vi "Module Loop.vi"(8 "error in (no error)":errorcluster, 11 "DAQmxAO in":refnum<class "DAQmxAO.lvclass">) -> (0 "error out":errorcluster, 3 "DAQmxAO out":refnum<class "DAQmxAO.lvclass">)   [LabVIEW 2023, in "VolatusDAQ.lvlib" / "DAQmxAO.lvclass"]
uses:
  DAQmxAO.lvclass
  DAQmxAO.lvclass/DAQmxAO.ctl
  Volatus/Module/Module.lvclass
  Volatus/MessageQ/MessageQ.lvclass/MessageQ.ctl
  messages/CmdAnalog/Class/Msg.lvclass/Msg.ctl
  Volatus/Module/Module.lvclass/Module.ctl
  messages/CmdAnalog/Data.ctl
  VolatusData/Scaling/Scaling.lvclass/Scaling.ctl
  messages/CmdAnalogMultiple/Class/Msg.lvclass
  messages/CmdAnalogMultiple/Class/Msg.lvclass/Msg.ctl
  <vilib>/DAQmx/write.llb/DAQmx Write (Analog 1D DBL NChan 1Samp).vi
  VolatusData/Send New Data (Array).vi
  Volatus/Module/Self Q.vi
  Volatus/MessageQ/Send.vi
  VolatusData/Scaling/Scale Channel (Scalar).vi
  Volatus/Module/Report Event.vi
  Volatus/Module/Format Num Array Cmd.vi
  VolatusData/Scaling/Polynomial Evaluate.vi
  VolatusData/Scaling/Expo Scale Value.vi
  <vilib>/AdvancedString/1D String Array to Delimited String.vi
  VolatusData/Scaling/Polynomial Remove Trailing Zeros.vi
  lv-vecto/Vecto/Group DBL/Group DBL.lvclass
  <vilib>/DAQmx/miscellaneous.llb/DAQmx Fill In Error Info.vi
  Volatus/VolatusAPI/Report Event.vi
  <vilib>/Utility/error.llb/Error Cluster From Error Code.vi
  VolatusData/Scaling/Scaling.lvclass
  messages/CmdAnalog/CmdAnalog.lvlib
  C:/dev/volatus/mts-volatus-super/libs/lv-volatus/Volatus/Module/Module.lvclass
  C:/dev/volatus/mts-volatus-super/libs/lv-volatus/VolatusDAQ/DAQmxAO/DAQmxAO.lvclass
  messages/CmdAnalogMultiple/Data.ctl
  messages/CmdAnalogMultiple/CmdAnalogMultiple.lvlib
  C:/dev/volatus/mts-volatus-super/libs/lv-volatus/messages/CmdAnalogMultiple/Class/Msg.lvclass
  C:/dev/volatus/mts-volatus-super/libs/lv-protoc/LV-Proto/Message/Message.lvclass
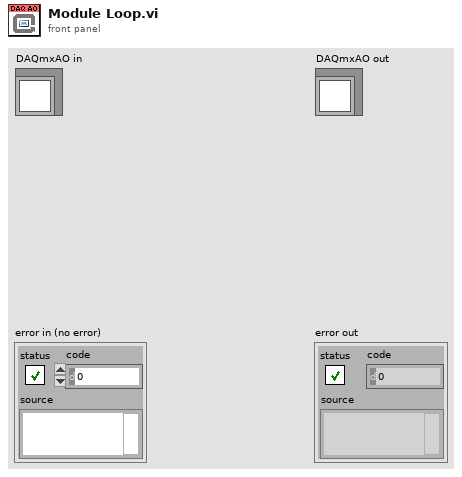
[diagram p1: front panel]
types:
  T1 = enum32{"Invalid", "Standard", "Closed", "Hidden", "Minimized", "Maximized"}
  T2 = typedef "CmdAnalogMultiple.lvlib/Data.ctl" = cluster{"values":T3[]}
  T3 = typedef "CmdAnalog.lvlib/Data.ctl" = cluster{"channel":string, "value":dbl}
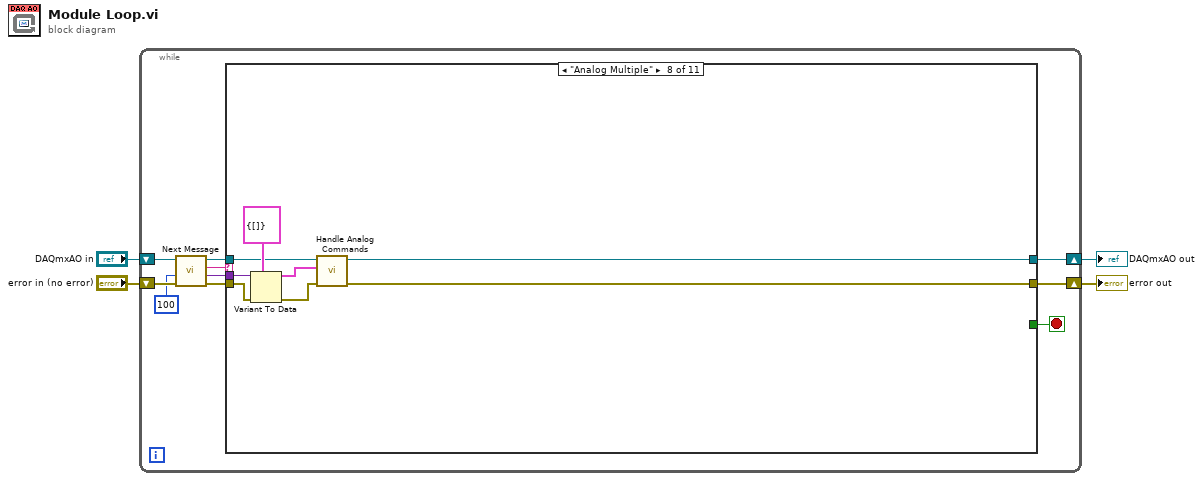
[diagram p0: block diagram]
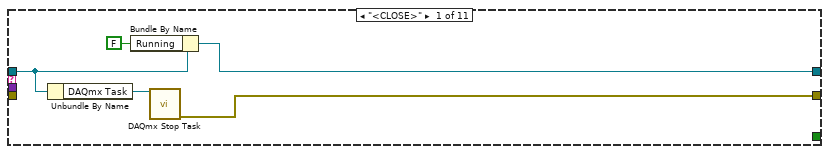
[diagram p2: hidden frame]
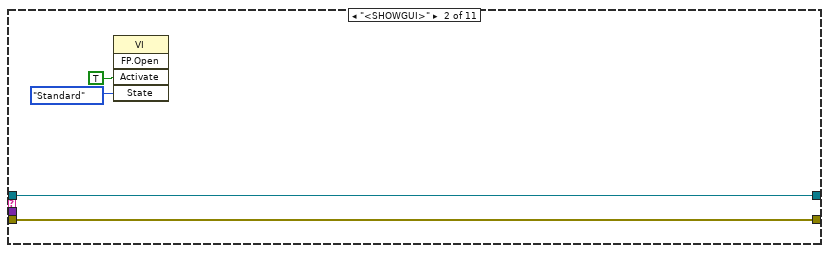
[diagram p3: hidden frame]
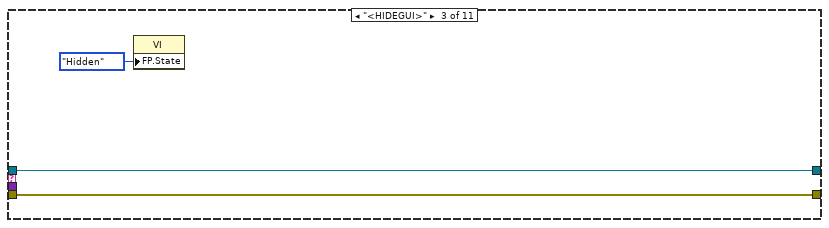
[diagram p4: hidden frame]
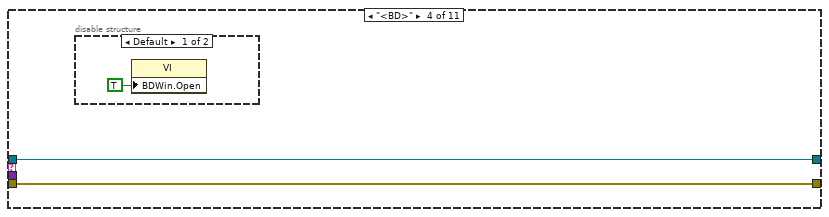
[diagram p5: hidden frame]
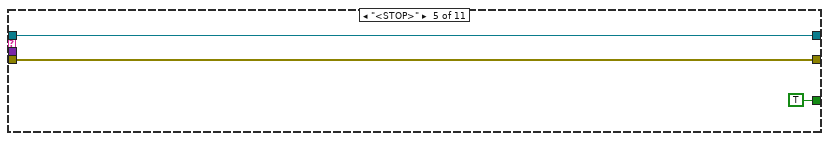
[diagram p7: hidden frame]
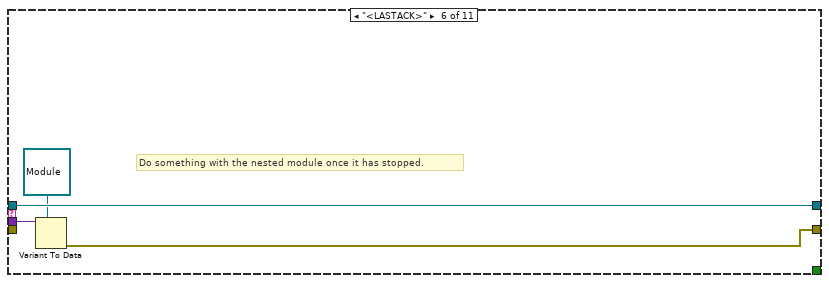
[diagram p8: hidden frame]
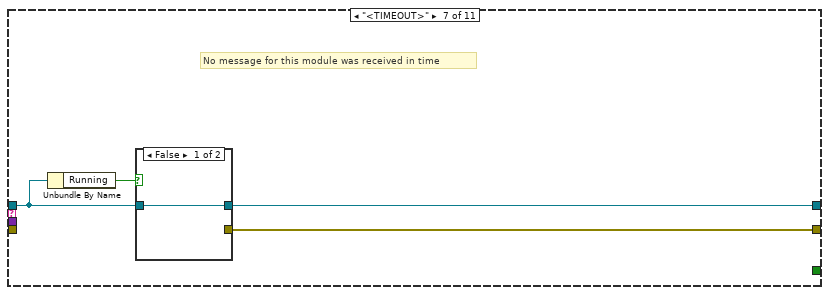
[diagram p9: hidden frame]
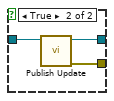
[diagram p10: hidden frame]
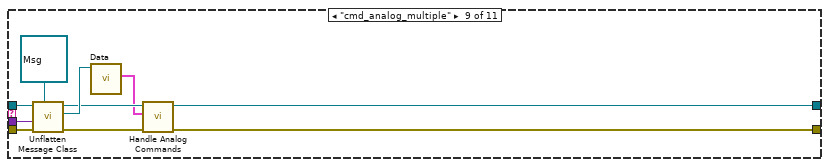
[diagram p11: hidden frame]
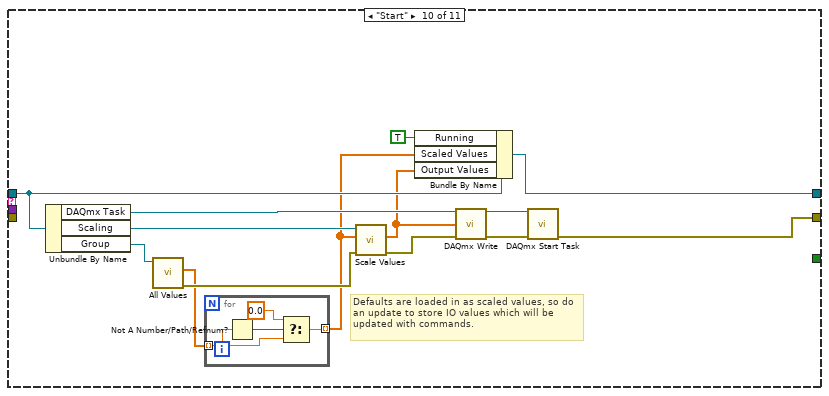
[diagram p12: hidden frame]
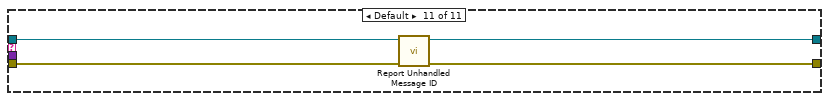
[diagram p13: hidden frame]
diagram:
  n1 = while {
    shift-right: [w9] -> w2
    shift-left: "DAQmxAO in" -> [w14]
    shift-right: [w8] -> w1
    shift-left: "error in (no error)" -> [w13]
    stop <- w7 stop-if-true
    n2 = call "Next Message.vi"("error in (no error)"=w13, "Timeout/Period ms (-1)"=100 ("Timeout ms (-1)"), "Module in"=w14) -> ("error out"=w12:errorcluster, "Data"=w6:variant, "ID"=w11:string, "Module out"=w10:refnum<class "DAQmxAO.lvclass">)  [unwired: 5 in]
    n3 = case shown="\"Analog Multiple\"" w11 {
      tunnel: w12 -> [_ w22 w25 w27 w31 _ _ w50 w62 _ w84]
      tunnel: w10 -> [w19 w23 w26 w28 w32 w36 w40 w49 w61 w75 w82]
      tunnel: [w17 w23 w26 w28 w32 w36 w39 w45 w53 w67 w81] -> w9
      tunnel: [w15 w22 w25 w27 w31 w33 w38 w46 w54 w64 w83] -> w8
      tunnel: [_ _ _ _ TRUE _ _ _ _ _ _] -> w7
      tunnel: w6 -> [_ _ _ _ _ w35 _ w52 w60 _ _]
      frame "<CLOSE>" {
        n4 = Unbundle By Name(w19) -> ("DAQmx Task"=w18:refnum<k21>)
        n5 = Bundle By Name(cluster=w19, "Running"=FALSE) -> (w17:refnum<class "DAQmxAO.lvclass">)
        n6 = call <vilib>:"DAQmx Stop Task.vi"("task/channels in"=w18) -> ("error out"=w15:errorcluster)  [unwired: 13 in, 1 out]
      }
      frame "<SHOWGUI>" {
        n7 = invoke class="VI" method="FP.Open"("Activate"=TRUE ("Activate?"), "State"=T1."Standard") -> ()  [unwired: 3 in, 5 out]
      }
      frame "<HIDEGUI>" {
        n8 = property class="VI"("FP.State"=T1."Hidden" ("Front Panel Window:State")) -> ()  [unwired: 2 in, 2 out]
      }
      frame "<BD>" {
        n9 = disable-structure shown="Default" {
          frame condition #0 (active) {
            n10 = property class="VI"("BDWin.Open"=TRUE ("Block Diagram Window:Open")) -> ()  [unwired: 2 in, 2 out]
          }
          frame condition #1 {
          }
        }
      }
      frame "<STOP>" {
      }
      frame "<LASTACK>" {
        # "Do something with the nested module once it has stopped."
        n11 = Variant To Data(type=refnum<class "Module.lvclass"> refnum ("Volatus:Module"), Variant=w35) -> (error out=w33:errorcluster)  [unwired: 1 in, 1 out]
      }
      frame "<TIMEOUT>" {
        # "No message for this module was received in time"
        n12 = Unbundle By Name(w40) -> ("Running"=w37:bool)
        n13 = case shown="False" w37 {
          tunnel: w40 -> [w41 w44]
          tunnel: [w41 w43] -> w39
          tunnel: [_ w42] -> w38
          frame False {
          }
          frame True {
            n14 = call "Publish Update.vi"("DAQmxAO in"=w44) -> ("error out"=w42:errorcluster, "DAQmxAO out"=w43:refnum<class "DAQmxAO.lvclass">)  [unwired: 9 in]
          }
        }
      }
      frame "Analog Multiple" {
        n15 = Variant To Data(error in=w50, type=T2 {"values"=[]} ("CmdAnalogMultiple"), Variant=w52) -> (data=w48:T2, error out=w47:errorcluster)
        n16 = call "Handle Analog Commands.vi"("error in (no error)"=w47, "Commands"=w48, "DAQmxAO in"=w49) -> ("error out"=w46:errorcluster, "DAQmxAO out"=w45:refnum<class "DAQmxAO.lvclass">)  [unwired: 7 in]
      }
      frame "cmd_analog_multiple" {
        n17 = call "Unflatten Message Class.vi"("Message Type"=refnum<class "Msg.lvclass"> refnum ("CmdAnalogMultiple.lvlib:Msg.lvclass"), "error in (no error)"=w62, "Data"=w60, "Module in"=w61) -> ("error out"=w55:errorcluster, "Message"=w58:refnum<class "Msg.lvclass">, "Module out"=w57:refnum<class "DAQmxAO.lvclass">)  [unwired: 4 in, 1 out]
        n18 = call "Data.vi"("PB Msg Template in"=w58) -> ("Data"=w56:T2)  [unwired: 8 in, 2 out]
        n19 = call "Handle Analog Commands.vi"("error in (no error)"=w55, "Commands"=w56, "DAQmxAO in"=w57) -> ("error out"=w54:errorcluster, "DAQmxAO out"=w53:refnum<class "DAQmxAO.lvclass">)  [unwired: 7 in]
      }
      frame "Start" {
        # "Defaults are loaded in as scaled values, so do an update to store IO values which will be updated with commands."
        n20 = Unbundle By Name(w75) -> ("DAQmx Task"=w72:refnum<k21>, "Scaling"=w73:refnum<class "Scaling.lvclass">, "Group"=w74:refnum<class "Group DBL.lvclass">)
        n21 = call "All Values.vi"("Group in"=w74) -> ("error out"=w76:errorcluster, "Scaled"=w69:dbl[])  [unwired: 6 in, 3 out]
        n22 = for {
          tunnel: w69 -> [w79] mode=indexing
          tunnel: [w77] -> w66 mode=indexing
          n23 = Not A Number/Path/Refnum?(number/path/refnum=w79) -> (NaN/Path/Refnum?=w80:bool)
          n24 = Select(t=0.0, s=w80, f=w79) -> (s? t:f=w77:dbl)
        }
        n25 = call "Scale Values.vi"("error in (no error)"=w76, "Values"=w66, "VolatusScaling in"=w73) -> ("error out"=w68:errorcluster, "Scaled Values"=w65:dbl[])  [unwired: 6 in, 1 out]
        n26 = Bundle By Name(cluster=w75, "Running"=TRUE, "Scaled Values"=w66, "Output Values"=w65) -> (w67:refnum<class "DAQmxAO.lvclass">)
        n27 = call-poly <vilib>:"DAQmx Write.vi"("task/channels in"=w72, "data"=w65, "error in"=w68) -> ("task out"=w71:refnum<k21>, "error out"=w70:errorcluster)  [unwired: 10 in, 1 out]
        n28 = call <vilib>:"DAQmx Start Task.vi"("task/channels in"=w71, "error in"=w70) -> ("error out"=w64:errorcluster)  [unwired: 12 in, 1 out]
      }
      frame Default {
        n29 = call "Report Unhandled Message ID.vi"("error in (no error)"=w84, "Module in"=w82) -> ("error out"=w83:errorcluster, "Module out"=w81:refnum<class "DAQmxAO.lvclass">)  [unwired: 8 in]
      }
    }
  }
  "error out" <- w1
  "DAQmxAO out" <- w2
